vi "Coord window-Add coord to list.vi"(11 "Coordinate list window refs":T1) -> (0 "error out":errorcluster, 2 "Number of rows":i32)   [LabVIEW 2020]
uses:
  Typedefs/Coordinate list window refs.ctl
  Globals/Coord window-Globals.vi
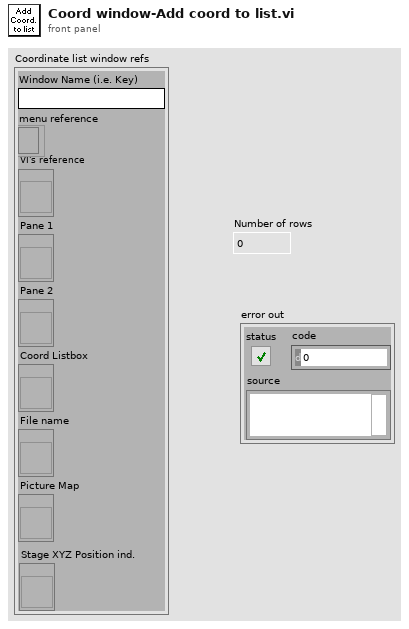
[diagram p1: front panel]
types:
  T1 = typedef "Coordinate list window refs.ctl" = cluster{"Window Name (i.e. Key)":string, "menu reference":refnum<k9>, "VI's reference":refnum<vi>, "Pane 1":refnum<vi>, "Pane 2":refnum<vi>, "Coord Listbox":refnum<vi>, "File name":refnum<vi>, "Picture Map":refnum<vi>, "Stage XYZ Position ind.":refnum<vi>}
  T2 = cluster{"Caption-Right button":string, "Caption-Left button":string, "Message to display":string, "Delay before close":u32, "Window Colour":u32, "Cancel button disabled?":enum8{"Enabled", "Disabled", "Disabled and Grayed Out"}}
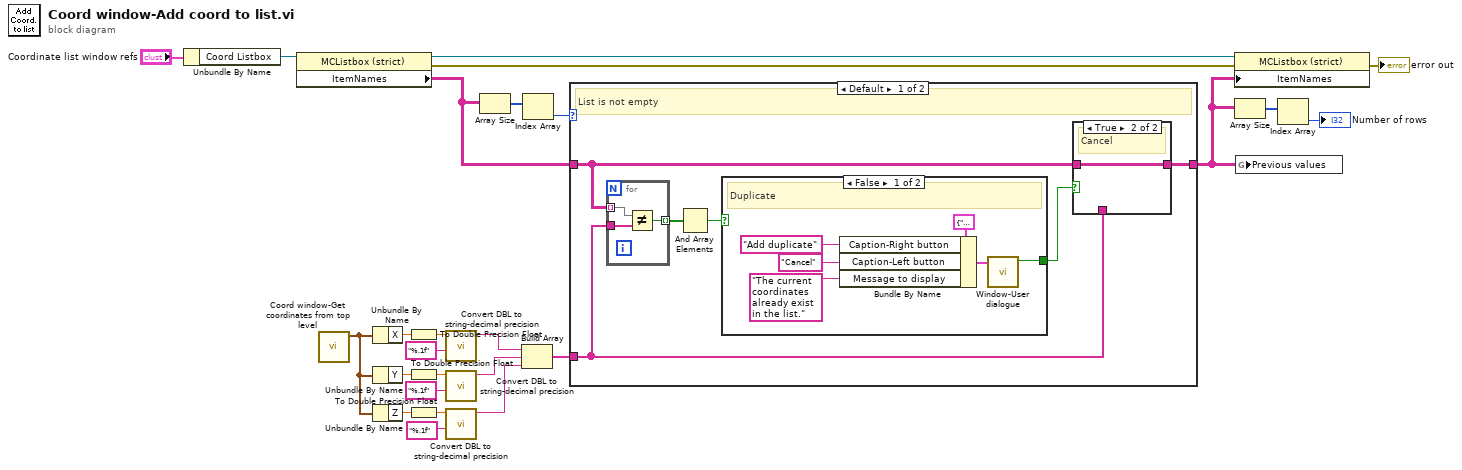
[diagram p0: block diagram]
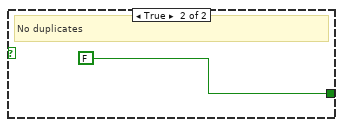
[diagram p2: hidden frame]
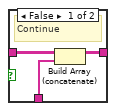
[diagram p3: hidden frame]
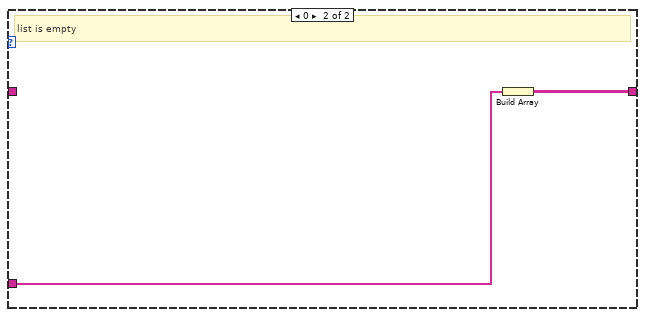
[diagram p4: hidden frame]
diagram:
  n1 = Unbundle By Name("Coordinate list window refs") -> ("Coord Listbox"=w19:refnum<vi>)
  n2 = property class="MCListbox (strict)"(reference=w19) -> (reference out=w23:refnum<vi>, error out=w21:errorcluster, "ItemNames"=w15:string[][])  [unwired: 1 in]
  n3 = call "Coord window-Get coordinates from top level.vi"() -> ("Coordinates"=w6:cluster{"X":sgl, "Y":sgl, "Z":sgl})  [unwired: 11 in]
  n4 = Unbundle By Name(w6) -> ("X"=w5:sgl)
  n5 = Unbundle By Name(w6) -> ("Y"=w7:sgl)
  n6 = Unbundle By Name(w6) -> ("Z"=w8:sgl)
  n7 = To Double Precision Float(number=w5) -> (double precision float=w12:dbl)
  n8 = To Double Precision Float(number=w7) -> (double precision float=w13:dbl)
  n9 = To Double Precision Float(number=w8) -> (double precision float=w14:dbl)
  n10 = call <userlib>:"Convert DBL to string-decimal precision.vi"("Format (%f)"="%.1f", "DBL Value"=w12) -> ("Converted to String"=w9:string)  [unwired: 9 in]
  n11 = call <userlib>:"Convert DBL to string-decimal precision.vi"("Format (%f)"="%.1f", "DBL Value"=w13) -> ("Converted to String"=w10:string)  [unwired: 9 in]
  n12 = call <userlib>:"Convert DBL to string-decimal precision.vi"("Format (%f)"="%.1f", "DBL Value"=w14) -> ("Converted to String"=w11:string)  [unwired: 9 in]
  n13 = Array Size(array=w15) -> (size(s)=w25:i32[])
  n14 = Build Array(w9, w10, w11) -> (w4:string[])
  n15 = Index Array(array=w25) -> (element=w24:i32)  [unwired: 1 in]
  n16 = case shown="Default" w24 {
    tunnel: w15 -> [w30 _]
    tunnel: w4 -> [w29 w47]
    tunnel: [w31 w46] -> w18
    frame Default {
      # "List is not empty"
      n17 = for {
        tunnel: w30 -> [w45] mode=indexing
        tunnel: w29 -> [w44]
        tunnel: [w43] -> w28 mode=indexing
        n18 = Not Equal?(x=w45, y=w44) -> (x != y?=w43:bool)
      }
      n19 = And Array Elements(Boolean array=w28) -> (logical AND=w27:bool)
      n20 = case shown="False" w27 {
        tunnel: [w32 FALSE] -> w26
        frame False {
          # "Duplicate"
          n21 = Bundle By Name(cluster=T2 {"Caption-Right button"="", "Caption-Left button"="", "Message to display"="", "Delay before close"=0, "Window Colour"=16448250, "Cancel button disabled?"=enum."Enabled"} ("Input cluster"), "Caption-Right button"="Add duplicate", "Caption-Left button"="Cancel", "Message to display"="The current coordinates already exist in the list.") -> (w33:T2)
          n22 = call "Window-User dialogue.vi"("Input cluster"=w33) -> ("Left Button (Cancel)"=w32:bool)  [unwired: 10 in]
        }
        frame True {
          # "No duplicates"
        }
      }
      n23 = case shown="True" w26 {
        tunnel: [w41 w42] -> w31
        tunnel: w30 -> [w40 w42]
        tunnel: w29 -> [w39 _]
        frame False {
          # "Continue"
          n24 = Build Array (concatenate)(w40, w39) -> (w41:string[][])
        }
        frame True {
          # "Cancel"
        }
      }
    }
    frame 0 {
      # "list is empty"
      n25 = Build Array(w47) -> (w46:string[][])
    }
  }
  n26 = property class="MCListbox (strict)"(reference=w23, error in=w21, "ItemNames"=w18) -> (error out=→"error out":errorcluster)  [unwired: 1 out]
  n27 = Array Size(array=w18) -> (size(s)=w17:i32[])
  n28 = global write "Coord window-Globals.vi" "Previous values"(w18) -> ()
  n29 = Index Array(array=w17) -> (element=→"Number of rows":i32)  [unwired: 1 in]
